vi "PM100D_GetRngIndex.vi"(5 "error in (no error)":errorcluster, 11 "VISA in":refnum<visa-resource-name>) -> (0 "error out":errorcluster, 1 "SensType":i32 min=0 max=5, 2 "Rng_Array":string[](array[string]), 3 "dup VISA session":refnum<visa-resource-name>, 4 "IndexOut":i32, 9 "AutoOut":bool)   [LabVIEW 2013]
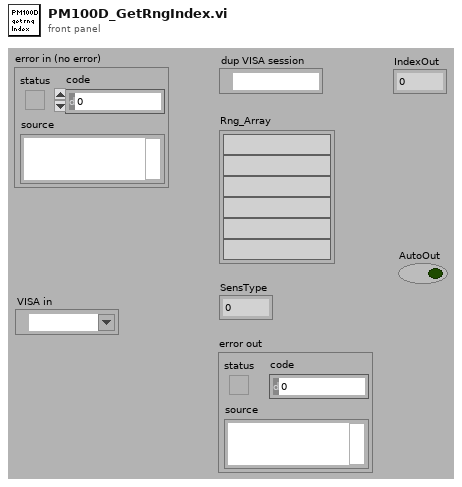
[diagram p1: front panel]
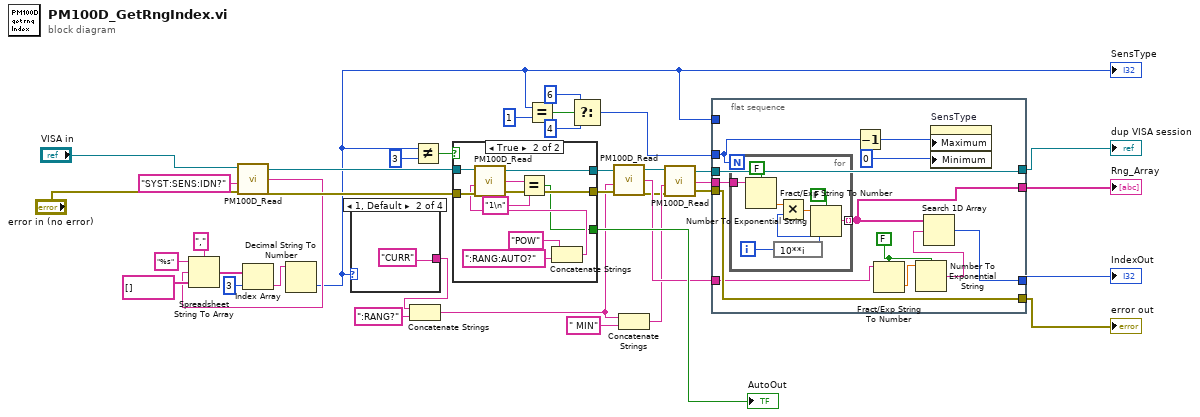
[diagram p0: block diagram]
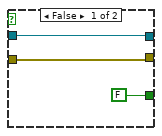
[diagram p2: hidden frame]
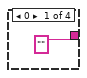
[diagram p3: hidden frame]
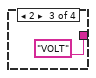
[diagram p4: hidden frame]
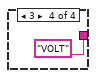
[diagram p5: hidden frame]
diagram:
  n1 = call "PM100D_Read.vi"("error in (no error)"="error in (no error)", "Command"="SYST:SENS:IDN?", "VISA in"="VISA in") -> ("error out"=w34:errorcluster, "ReadValue"=w25:string, "VISA out"=w32:refnum<visa-resource-name>)  [unwired: 1 in]
  n2 = Spreadsheet String To Array(delimiter (Tab)=",", format string="%s", spreadsheet string=w25, array type (2D Dbl)=string[] [] ("Rng_Array")) -> (array=w27:string[])
  n3 = Index Array(array=w27, index=3) -> (element=w30:string)
  n4 = Decimal String To Number(string=w30) -> (number=w2:i32)  [unwired: 2 in, 1 out]
  "SensType" <- w2
  n5 = case shown="1, Default" w2 {
    tunnel: ["" "CURR" "VOLT" "VOLT"] -> w19
    frame 0 {
    }
    frame 1, Default {
    }
    frame 2 {
    }
    frame 3 {
    }
  }
  n6 = Concatenate Strings(w19, ":RANG?" ("string")) -> (w7:string)
  n7 = Not Equal?(x=w2, y=3) -> (x != y?=w37:bool)
  n8 = case shown="True" w37 {
    tunnel: w32 -> [w45 w55]
    tunnel: [w45 w54] -> w33
    tunnel: w34 -> [w44 w53]
    tunnel: [w44 w52] -> w35
    tunnel: [FALSE w46] -> w38
    frame False {
    }
    frame True {
      n9 = Concatenate Strings("POW" ("string"), ":RANG:AUTO?" ("string")) -> (w51:string)
      n10 = call "PM100D_Read.vi"("error in (no error)"=w53, "Command"=w51, "VISA in"=w55) -> ("error out"=w52:errorcluster, "ReadValue"=w48:string, "VISA out"=w54:refnum<visa-resource-name>)  [unwired: 1 in]
      n11 = Equal?(x=w48, y="1\n") -> (x = y?=w46:bool)
    }
  }
  "AutoOut" <- w38
  n12 = Equal?(x=w2, y=1) -> (x = y?=w21:bool)
  n13 = Select(t=6, s=w21, f=4) -> (s? t:f=w10:i32)
  n14 = call "PM100D_Read.vi"("error in (no error)"=w35, "Command"=w7, "VISA in"=w33) -> ("error out"=w5:errorcluster, "ReadValue"=w16:string, "VISA out"=w4:refnum<visa-resource-name>)  [unwired: 1 in]
  n15 = Concatenate Strings(w7, " MIN" ("string")) -> (w8:string)
  n16 = call "PM100D_Read.vi"("error in (no error)"=w5, "Command"=w8, "VISA in"=w4) -> ("error out"=w14:errorcluster, "ReadValue"=w15:string, "VISA out"=w13:refnum<visa-resource-name>)  [unwired: 1 in]
  n17 = flat-sequence {
    tunnel: w10 -> [w59]
    tunnel: w13 -> [w67]
    tunnel: [w67] -> w17
    tunnel: [w66] -> w18
    tunnel: w14 -> [w66]
    tunnel: w15 -> [w65]
    tunnel: w16 -> [w64]
    tunnel: [w60] -> w3
    tunnel: [w58] -> w1
    tunnel: w2 -> [_]
    frame #0 {
      w62 = FALSE ("use system decimal point (T)")
      n18 = for {
        N: w59 -> [_]
        tunnel: w65 -> [w74]
        tunnel: [w68] -> w60 mode=indexing
        i -> [w75]
        n19 = Fract/Exp String To Number(use system decimal point (T)=FALSE, string=w74) -> (number=w73:dbl)  [unwired: 2 in, 1 out]
        n20 = expression code="10**i"(w75) -> (w72:i32)
        n21 = Multiply(x=w73, y=w72) -> (x*y=w70:dbl)
        n22 = Number To Exponential String(number=w70, 1:FALSE ("use system decimal point (T)")) -> (E-format string=w68:string)  [unwired: 2 in]
      }
      n23 = Decrement(x=w59) -> (x-1=w57:i32)
      n24 = Fract/Exp String To Number(use system decimal point (T)=w62, string=w64) -> (number=w63:dbl)  [unwired: 2 in, 1 out]
      n25 = Number To Exponential String(number=w63, 1:w62) -> (E-format string=w61:string)  [unwired: 2 in]
      n26 = Search 1D Array(1D array=w60, element=w61) -> (index of element=w58:i32)  [unwired: 1 in]
      n27 = property on="SensType" class="DigNum (strict)"("Maximum"=w57, "Minimum"=0) -> ()  [unwired: 2 in, 2 out]
    }
  }
  "Rng_Array" <- w3
  "error out" <- w18
  "dup VISA session" <- w17
  "IndexOut" <- w1
